vi "Add_Destination.vi"(7 "parent tag":string, 8 "error in (no error)":errorcluster, 9 "Destinations in":refnum<class "IB_Destination.lvclass">[](array[class]), 10 "new destination in":refnum<class "IB_Destination.lvclass">, 11 "IB_DestTree in":refnum<class "IB_Tree_Dest.lvclass">) -> (0 "error out":errorcluster, 1 "Destinations out":refnum<class "IB_Destination.lvclass">[](array[class]), 2 "duplicate?":bool, 3 "IB_DestTree out":refnum<class "IB_Tree_Dest.lvclass">, 5 "edits":T1[](array[typedef]))   [LabVIEW 2020, in "IB_Tree_Dest.lvclass"]
uses:
  <vilib>/AppBuilder/IB_Classes/Tree_Dest/IB_Tree_Dest.lvclass
  <vilib>/AppBuilder/IB_Classes/Tree_Dest/IB_Tree_Dest.lvclass/IB_Tree_Dest.ctl
  <vilib>/AppBuilder/IB_Classes/Destination/IB_Destination.lvclass
  <vilib>/AppBuilder/IB_Classes/Tree/IB_Tree.lvclass
  <vilib>/AppBuilder/IB_Classes/Tree_Dest/destEdits_operation.ctl
  <vilib>/AppBuilder/IB_Classes/Tree_Dest/destEdits_edit.ctl
  <vilib>/AppBuilder/IB_Classes/Tree_Dest/destEdits_add.ctl
  e:/builds/penguin/labview/branches/2020/dev/dist/vi.lib/AppBuilder/IB_Classes/Tree/IB_Tree.lvclass
  e:/builds/penguin/labview/branches/2020/dev/dist/vi.lib/AppBuilder/IB_Classes/Tree_Dest/IB_Tree_Dest.lvclass
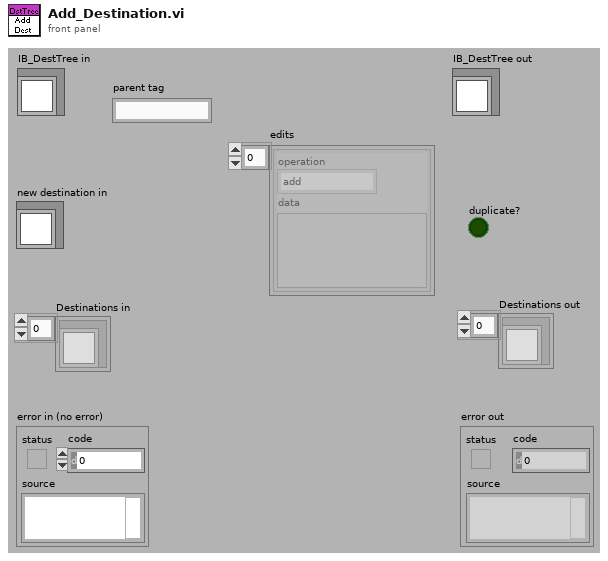
[diagram p1: front panel]
types:
  T1 = typedef "destEdits_edit.ctl" = cluster{"operation":T2, "data":variant}
  T2 = typedef "destEdits_operation.ctl" = enum16{"add", "remove", "rename", "sort children", "default dir changed"}
  T3 = typedef "destEdits_add.ctl" = cluster{"parent tag":string, "child tag":string, "left cell string":string, "symbol index":i32}
  T4 = typedef "IB_Destination.ctl" = cluster{"name":string, "unlock":bool, "parentTag":string, "destTag":string, "eng_installPath":string}
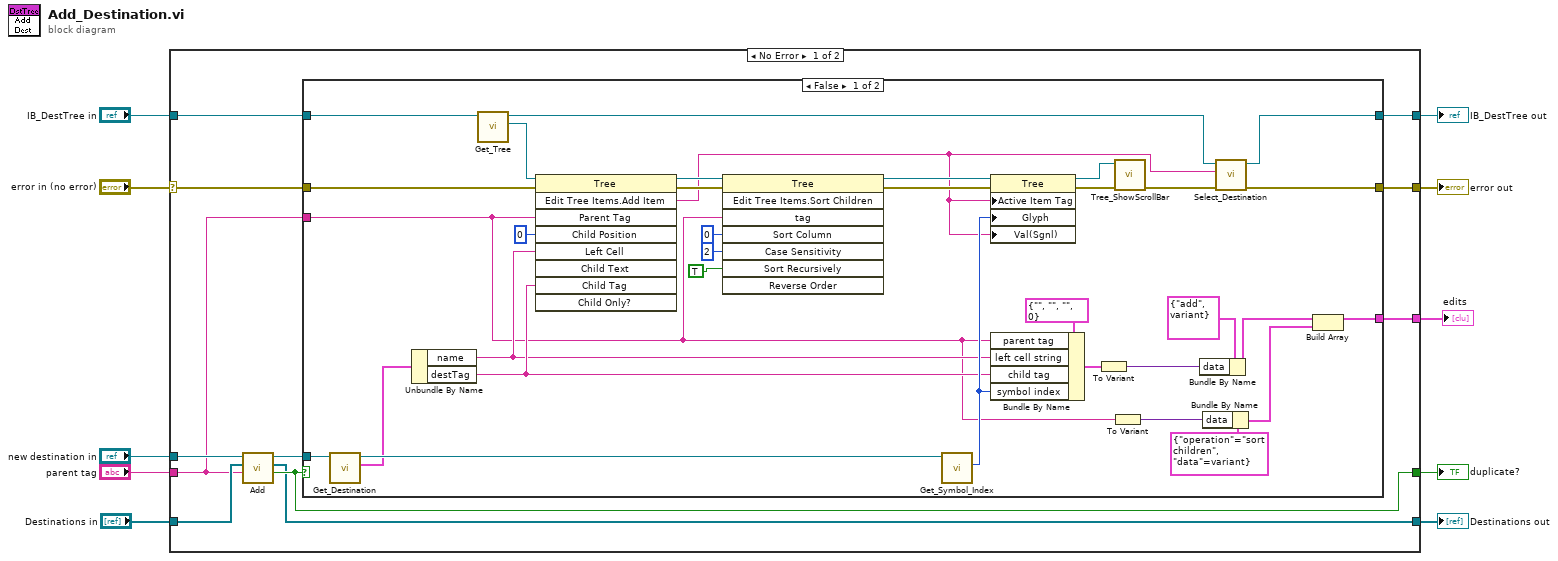
[diagram p0: block diagram]
diagram:
  n1 = case shown="No Error" "error in (no error)" {
    selector: "error in (no error)" -> [w14 w60]
    tunnel: [w18 w60] -> w9
    tunnel: [w19 w59] -> w7
    tunnel: "IB_DestTree in" -> [w21 w59]
    tunnel: "new destination in" -> [w17 _]
    tunnel: "parent tag" -> [w15 _]
    tunnel: [w20 _] -> w1
    tunnel: "Destinations in" -> [w16 w58]
    tunnel: [w11 w58] -> w3
    tunnel: [w12 _] -> w2
    frame No Error {
      n2 = call-dynamic "Add.vi"("parent tag"=w15, "Destinations in"=w16, "IB_Destination in"=w17) -> ("duplicate?"=w12:bool, "Destinations out"=w11:refnum<class "IB_Destination.lvclass">[], "IB_Destination out"=w13:refnum<class "IB_Destination.lvclass">)  [unwired: 1 in, 5 out]
      n3 = case shown="False" w12 {
        tunnel: w21 -> [w55 w57]
        tunnel: [w22 _] -> w20
        tunnel: [w46 w57] -> w19
        tunnel: [w44 w56] -> w18
        tunnel: w15 -> [w26 _]
        tunnel: w14 -> [w43 w56]
        tunnel: w13 -> [w41 _]
        frame False {
          n4 = call <vilib>:"Get_Destination.vi"("IB_Destination in"=w41) -> ("data"=w39:T4, "IB_Destination out"=w40:refnum<class "IB_Destination.lvclass">)  [unwired: 1 in, 8 out]
          n5 = Unbundle By Name(w39) -> ("name"=w37:string, "destTag"=w38:string)
          n6 = call <vilib>:"Get_Tree.vi"("IB_Tree in"=w55) -> ("ctl"=w42:refnum<vi>, "IB_Tree out"=w47:refnum<class "IB_Tree_Dest.lvclass">)  [unwired: 1 in, 8 out]
          n7 = invoke class="Tree" method="Edit Tree Items.Add Item"(reference=w42, error in=w43, "Parent Tag"=w26, "Child Position"=0, "Left Cell"=w37, "Child Tag"=w38) -> (reference out=w35:refnum<vi>, error out=w32:errorcluster, "Edit Tree Items:Add Item"=w31:string)  [unwired: 3 in, 6 out]
          n8 = invoke class="Tree" method="Edit Tree Items.Sort Children"(reference=w35, error in=w32, "tag"=w26, "Sort Column"=0, "Case Sensitivity"=2, "Sort Recursively"=TRUE ("Sort Recursively?")) -> (reference out=w34:refnum<vi>, error out=w33:errorcluster)  [unwired: 2 in, 6 out]
          n9 = call-dynamic "Get_Symbol_Index.vi"("IB_Destination in"=w40) -> ("symbol index"=w48:i32)  [unwired: 1 in, 9 out]
          n10 = property class="Tree"(reference=w34, error in=w33, "Active Item Tag"=w31, "Glyph"=w48, "Val(Sgnl)"=w31) -> (reference out=w54:refnum<vi>, error out=w53:errorcluster)
          n11 = Bundle By Name(cluster=T3 {"parent tag"="", "child tag"="", "left cell string"="", "symbol index"=0} ("add"), "parent tag"=w26, "left cell string"=w37, "child tag"=w38, "symbol index"=w48) -> (w49:T3)
          n12 = To Variant(anything=w49) -> (Variant=w50:variant)
          n13 = To Variant(anything=w26) -> (Variant=w25:variant)
          n14 = call <vilib>:"Tree_ShowScrollBar.vi"("error in (no error)"=w53, "Tree"=w54) -> ("error out"=w45:errorcluster)  [unwired: 9 out]
          n15 = Bundle By Name(cluster=T1 {"operation"=enum."add", "data"=variant} ("edit"), "data"=w50) -> (w23:T1)
          n16 = Bundle By Name(cluster=T1 {"operation"=enum."sort children", "data"=variant} ("edit"), "data"=w25) -> (w24:T1)
          n17 = call <vilib>:"Select_Destination.vi"("error in (no error)"=w45, "destTag"=w31, "IB_DestTree in"=w47) -> ("error out"=w44:errorcluster, "IB_DestTree out"=w46:refnum<class "IB_Tree_Dest.lvclass">)  [unwired: 7 out]
          n18 = Build Array(w23, w24) -> (w22:T1[])
        }
        frame True {
        }
      }
    }
    frame Error {
    }
  }
  "error out" <- w9
  "IB_DestTree out" <- w7
  "Destinations out" <- w3
  "duplicate?" <- w2
  "edits" <- w1
